vi "Vision Processing.vi"(4 "error in (no error)":errorcluster, 7 "Image Size":T1=enum."320x240") -> ()   [LabVIEW 2017]
doc: "This VI runs in parallel to other tasks. It gets images from the camera, processes them for color or shape and use that information to affect robot behavior."
uses:
  <vilib>/Rock Robotics/WPI/Camera/WPI_CameraImageSize.ctl
  Robot Global Data.vi
  <vilib>/Rock Robotics/WPI/Camera/WPI_CameraWhite Balance Values.ctl
  <vilib>/Rock Robotics/WPI/Camera/WPI_CameraExposure Values.ctl
  <vilib>/Rock Robotics/WPI/Camera/WPI_CameraFrameRate.ctl
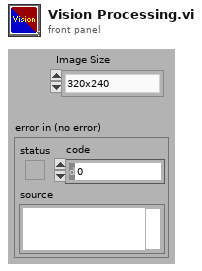
[diagram p1: front panel]
types:
  T1 = typedef "WPI_CameraImageSize.ctl" = enum16{"640x480", "320x240", "160x120", "Custom"}
  T2 = typedef "Image Type" = u32
  T3 = typedef "WPI_CameraFrameRate.ctl" = u32
  T4 = typedef "WPI_CameraExposure Values.ctl" = enum16{"Auto", "Flicker-free 50 Hz", "Flicker-free 60 Hz", "Hold current", "Custom"}
  T5 = typedef "WPI_CameraWhite Balance Values.ctl" = enum16{"Auto", "Fixed indoor", "Fixed outdoor 1", "Fixed outdoor 2", "Fixed fluorescent 1", "Fixed fluorescent 2", "Hold current", "Custom"}
  T6 = typedef "WPI_CameraDevRef.ctl" = cluster{"Camera Address":string, "CameraStatus":errorcluster}
  T7 = typedef "IMAQ Image.ctl" = refnum<image>
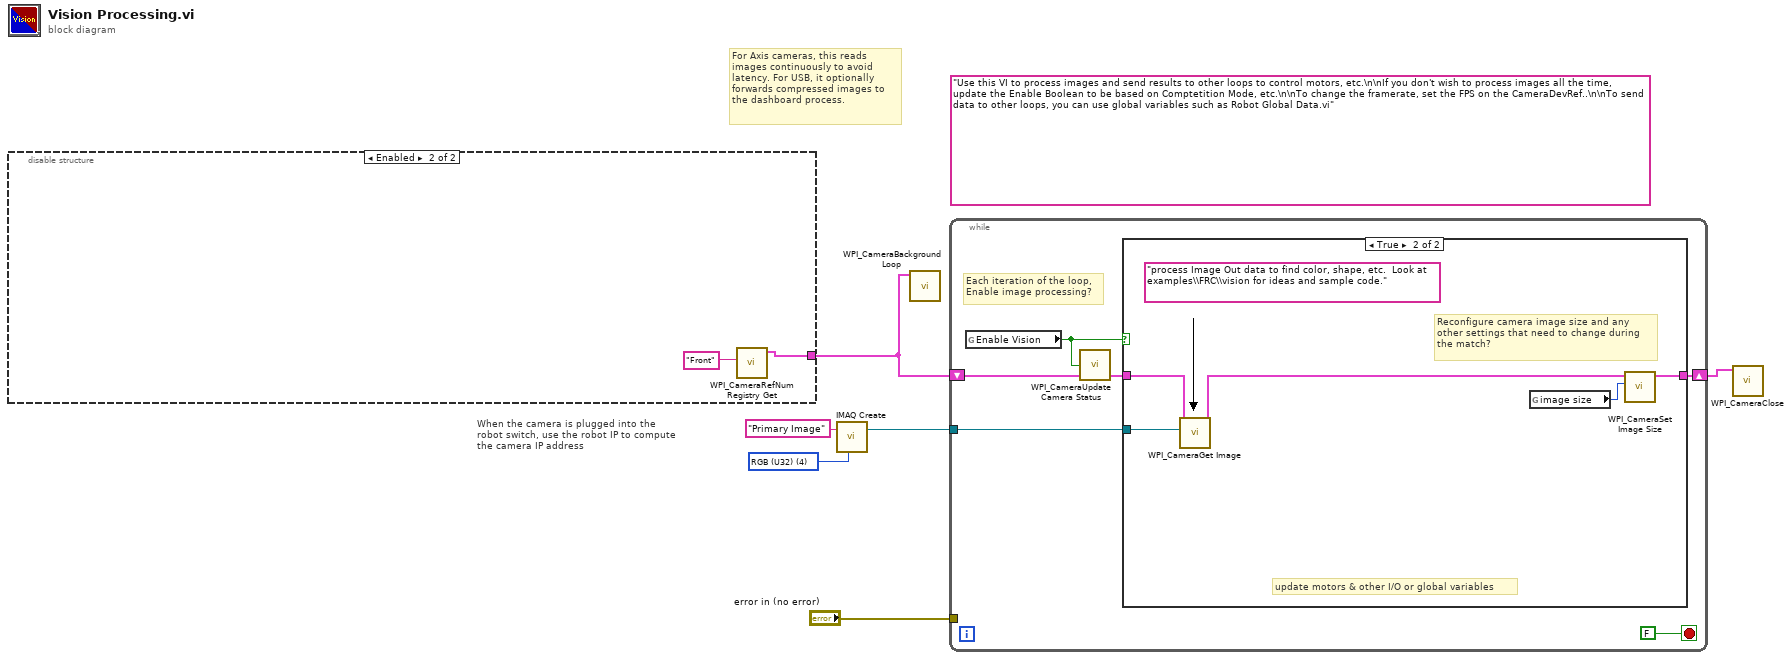
[diagram p0: block diagram]
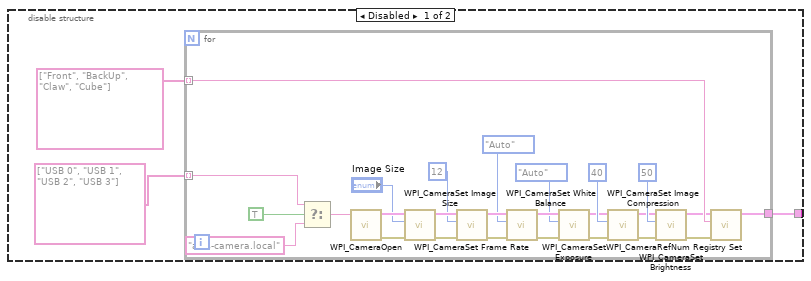
[diagram p2: hidden frame]
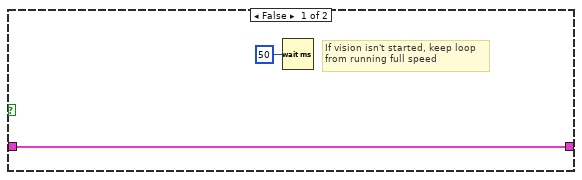
[diagram p3: hidden frame]
diagram:
  (unwired) "Use this VI to process images and send results to other loops to control motors, etc.\n\nIf you don't wish to process images all the time, update the Enable Boolean to be based on Comptetition Mode, etc.\n\nTo change the framerate, set the FPS on the CameraDevRef..\n\nTo send data to other loops, you can use global variables such as Robot Global Data.vi"
  w6 = T2 4 items=["Grayscale (U8)", "Grayscale (I16)", "Grayscale (SGL)", "Complex (CSG)", "RGB (U32)", "HSL (U32)", "RGB (U64)"] ("Image Type")
  # "When the camera is plugged into the\nrobot switch, use the robot IP to compute\nthe camera IP address"
  # "For Axis cameras, this reads\nimages continuously to avoid\nlatency. For USB, it optionally\nforwards compressed images to\nthe dashboard process."
  n1 = disable-structure shown="Enabled" {
    disable-tunnel: [w8 w37] -> w3
    frame Disabled {
      n2 = for {
        tunnel: string[] ["Front", "BackUp", "Claw", "Cube"] ("refnum name") -> [w35] mode=indexing
        tunnel: [w15] -> w8
        tunnel: string[] ["USB 0", "USB 1", "USB 2", "USB 3"] ("format string") -> [w13] mode=indexing
        n3 = Select(t=w13, s=TRUE ("dot notation? (F)"), f="axis-camera.local" ("format string")) -> (s? t:f=w11:string)
        n4 = call <vilib>:"WPI_CameraOpen.vi"("Camera Address"=w11) -> ("error out"=w26:errorcluster, "CameraDevRef"=w27:T6)  [unwired: 1 in, 8 out]
        n5 = call <vilib>:"WPI_CameraSet Image Size.vi"("error in (no error)"=w26, "Image Size"="Image Size", "CameraDevRef"=w27) -> ("error out"=w25:errorcluster, "CameraDevRef Out"=w28:T6)  [unwired: 1 in, 6 out]
        n6 = call <vilib>:"WPI_CameraSet Frame Rate.vi"("error in (no error)"=w25, "Frame Rate (fps)"=T3 12, "CameraDevRef"=w28) -> ("error out"=w24:errorcluster, "CameraDevRef Out"=w30:T6)  [unwired: 7 out]
        n7 = call <vilib>:"WPI_CameraSet White Balance.vi"("error in (no error)"=w24, "White Balance"=WPI_CameraWhite_Balance_Values."Auto", "CameraDevRef"=w30) -> ("error out"=w23:errorcluster, "CameraDevRef Out"=w29:T6)  [unwired: 1 in, 6 out]
        n8 = call <vilib>:"WPI_CameraSet Exposure.vi"("error in (no error)"=w23, "Exposure"=WPI_CameraExposure_Values."Auto", "CameraDevRef"=w29) -> ("error out"=w22:errorcluster, "CameraDevRef Out"=w32:T6)  [unwired: 1 in, 6 out]
        n9 = call <vilib>:"WPI_CameraSet Image Compression.vi"("error in (no error)"=w22, "Compression"=40, "CameraDevRef"=w32) -> ("error out"=w21:errorcluster, "CameraDevRef Out"=w31:T6)  [unwired: 7 out]
        n10 = call <vilib>:"WPI_CameraSet Brightness.vi"("error in (no error)"=w21, "Brightness"=50, "CameraDevRef"=w31) -> ("error out"=w19:errorcluster, "CameraDevRef Out"=w20:T6)  [unwired: 1 in, 6 out]
        n11 = call <vilib>:"WPI_CameraRefNum Registry Set.vi"("error in (no error)"=w19, "refnum name"=w35, "CameraDevRef"=w20) -> ("CameraDevRef"=w15:T6)  [unwired: 1 in, 7 out]
      }
    }
    frame Enabled {
      n12 = call <vilib>:"WPI_CameraRefNum Registry Get.vi"("refnum name"="Front") -> ("CameraDevRef"=w37:T6)  [unwired: 9 in, 1 out]
    }
  }
  n13 = call "IMAQ Create"("Image Name"="Primary Image", "Image Type"=w6) -> ("New Image"=w4:T7)  [unwired: 2 in, 2 out]
  n14 = call <vilib>:"WPI_CameraBackground Loop.vi"("CameraDevRef"=w3) -> ()  [unwired: 11 in]
  n15 = while {
    shift-right: [w42] -> w2
    shift-left: w3 -> [w40]
    tunnel: w4 -> [w41]
    tunnel: "error in (no error)" -> [_]
    stop <- FALSE stop-if-true
    # "Each iteration of the loop,\nEnable image processing?"
    n16 = global read "Robot Global Data.vi" "Enable Vision"() -> (w38:bool)
    n17 = call <vilib>:"WPI_CameraUpdate Camera Status.vi"("CameraDevRef In"=w40, "Enable Vision"=w38) -> ("CameraDevRef Out"=w39:T6)  [unwired: 3 in]
    n18 = case shown="True" w38 {
      tunnel: w41 -> [_ w49]
      tunnel: [w45 w50] -> w42
      tunnel: w39 -> [w45 w47]
      frame False {
        # "If vision isn't started, keep loop\nfrom running full speed"
        n19 = Wait (ms)(milliseconds to wait=u32 50) -> ()  [unwired: 1 out]
      }
      frame True {
        (unwired) "process Image Out data to find color, shape, etc.  Look at examples\\FRC\\vision for ideas and sample code."
        # "update motors & other I/O or global variables"
        # "Reconfigure camera image size and any\nother settings that need to change during\nthe match?"
        n20 = call <vilib>:"WPI_CameraGet Image.vi"("Image"=w49, "CameraDevRef"=w47) -> ("CameraDevRef Out"=w46:T6)  [unwired: 1 in, 8 out]
        n21 = global read "Robot Global Data.vi" "image size"() -> (w48:T1)
        n22 = call <vilib>:"WPI_CameraSet Image Size.vi"("Image Size"=w48, "CameraDevRef"=w46) -> ("CameraDevRef Out"=w50:T6)  [unwired: 2 in, 7 out]
      }
    }
  }
  n23 = call <vilib>:"WPI_CameraClose.vi"("CameraDevRef"=w2) -> ()  [unwired: 1 in, 10 out]
